vi "JSON to LVObject - Descendant Class And JSON Object With All Fields - Returns Descendant Class With All Fields Set.vi"() -> ()   [LabVIEW 2017, in "Generic Object Serializer Tests.lvlib"]
uses:
  Generic Object Serializer Tests.lvlib
  Generic Object Serializer/Generic Object Serializer.lvclass
  Temperature Forecast/Temperature Forecast.lvclass
  <vilib>/addons/_JKI Toolkits/Caraya/classes/Assert/Assert Equal Value and Type_Variant.vi
  <vilib>/addons/_JKI Toolkits/Caraya/classes/Test/Test.lvclass
  <vilib>/addons/_JKI Toolkits/Caraya/classes/Assert/Assert.lvclass
panel:
  out "error out":errorcluster
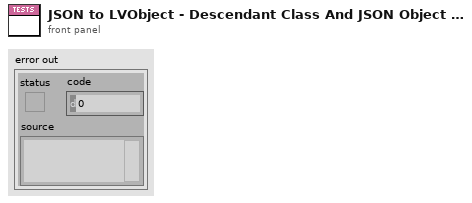
[diagram p1: front panel]
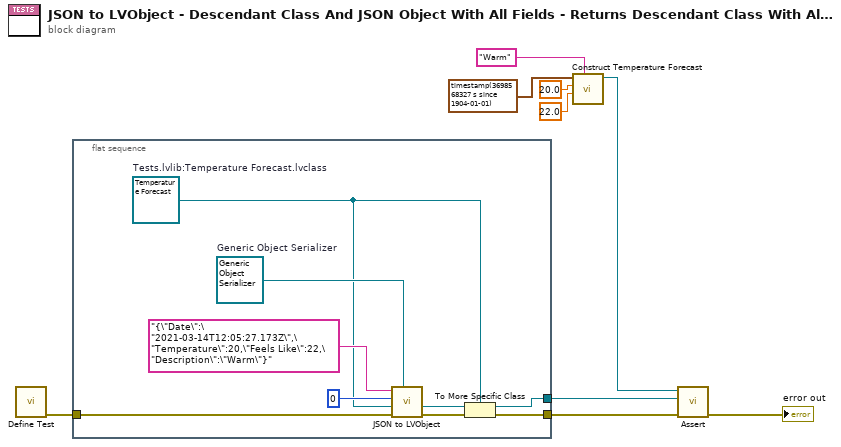
[diagram p0: block diagram]
diagram:
  n1 = call <vilib>:"Define Test.vi"() -> ("error out"=w9:errorcluster)  [unwired: 11 in]
  n2 = flat-sequence {
    tunnel: w9 -> [w17]
    tunnel: [w13] -> w8
    tunnel: [w10] -> w7
    frame #0 {
      w11 = refnum<class "Temperature Forecast.lvclass"> refnum  # Tests.lvlib:Temperature Forecast.lvclass
      w18 = refnum<class "Generic Object Serializer.lvclass"> refnum  # Generic Object Serializer
      n3 = call-dynamic "JSON to LVObject.vi"("LVClass Serializer"=w18, "error in (no error)"=w17, "Object Type"=w11, "Offset"=0, "JSON"="{\"Date\":\"2021-03-14T12:05:27.173Z\",\"Temperature\":20,\"Feels Like\":22,\"Description\":\"Warm\"}") -> ("error out"=w16:errorcluster, "Object"=w12:refnum<class>)  [unwired: 5 in]
      n4 = To More Specific Class(target class=w11, reference=w12, error in=w16) -> (specific class reference=w10:refnum<class "Temperature Forecast.lvclass">, error out=w13:errorcluster)
    }
  }
  n5 = call "Construct Temperature Forecast.vi"("Description"="Warm", "Feels Like [°C]"=22.0, "Temperature [°C]"=20.0, "Date"=timestamp(3698568327.173 s since 1904-01-01)) -> ("Temperature Forecast"=w5:refnum<class "Temperature Forecast.lvclass">)  [unwired: 6 in, 1 out]
  n6 = call-poly <vilib>:"Assert.vi"("error in (no error)"=w8, "Y"=w7, "X"=w5) -> ("error out"=→"error out":errorcluster)  [unwired: 8 in]
